vi "to-bool.vi"(1 "register":u16) -> (0 "簇":T1)   [LabVIEW 2015]
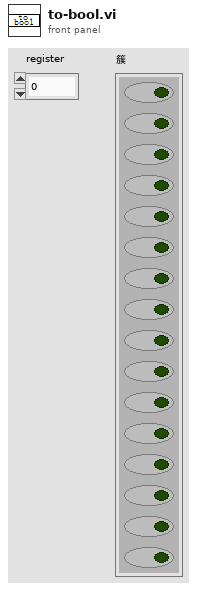
[diagram p1: front panel]
types:
  T1 = cluster{bool, bool, bool, bool, bool, bool, bool, bool, bool, bool, bool, bool, bool, bool, bool, bool}
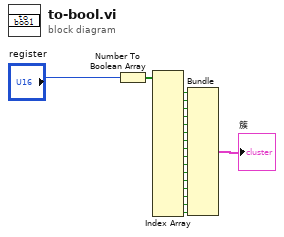
[diagram p0: block diagram]
diagram:
  n1 = Number To Boolean Array(number="register") -> (Boolean array=w2:bool[])
  n2 = Index Array(array=w2) -> (element #1=w3:bool, element #2=w4:bool, element #3=w5:bool, element #4=w6:bool, element #5=w7:bool, element #6=w8:bool, element #7=w9:bool, element #8=w10:bool, element #9=w11:bool, element #10=w12:bool, element #11=w13:bool, element #12=w14:bool, element #13=w15:bool, element #14=w16:bool, element #15=w17:bool, element #16=w18:bool)  [unwired: 16 in]
  n3 = Bundle(w3, w4, w5, w6, w7, w8, w9, w10, w11, w12, w13, w14, w15, w16, w17, w18) -> (→"簇":T1)  [unwired: 1 in]
